vi "End.vi"(8 "error in (no error)":errorcluster, 11 "PublisherGS in":refnum<class "PublisherGS.lvclass">) -> (0 "error out":errorcluster, 3 "PublisherGS out":refnum<class "PublisherGS.lvclass">)   [LabVIEW 2018, in "PublisherGS.lvclass"]
uses:
  PublisherGS.lvclass
  Client/Client.lvclass
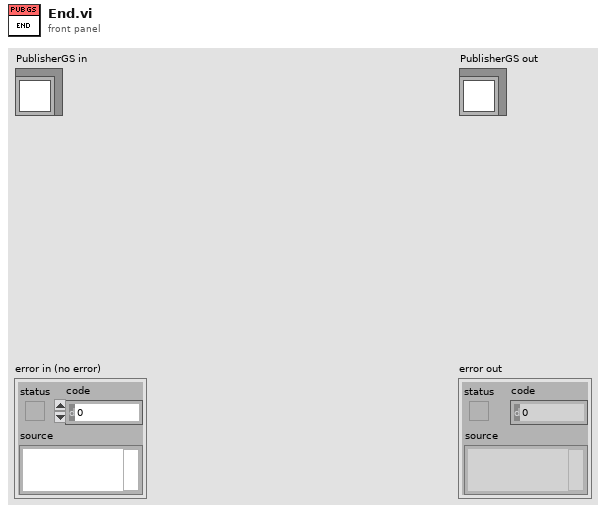
[diagram p1: front panel]
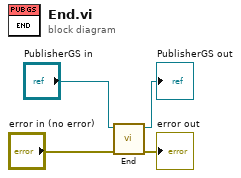
[diagram p0: block diagram]
diagram:
  n1 = call-parent "End.vi"("error in (no error)"="error in (no error)", "Client in"="PublisherGS in") -> ("error out"=→"error out":errorcluster, "Client out"=→"PublisherGS out":refnum<class "PublisherGS.lvclass">)  [unwired: 8 in]
